vi "Make Deployable VI Path.vi"(1 "instance path":path) -> (0 "deployable path":path)   [LabVIEW 2020, in "NI_TargetHelper.lvlib"]
uses:
  <vilib>/TargetSupport/NI_TargetHelper/NI_TargetHelper.lvlib
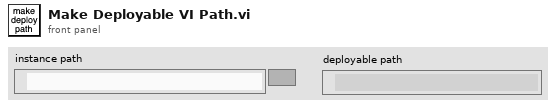
[diagram p1: front panel]
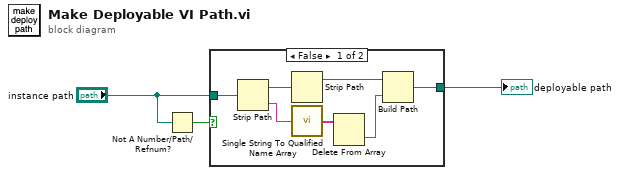
[diagram p0: block diagram]
diagram:
  n1 = Not A Number/Path/Refnum?(number/path/refnum="instance path") -> (NaN/Path/Refnum?=w2:bool)
  n2 = case shown="False" w2 {
    tunnel: "instance path" -> [w5 w11]
    tunnel: [w4 w11] -> w3
    frame False {
      n3 = Strip Path(path=w5) -> (stripped path=w7:path, name=w8:string)
      n4 = Strip Path(path=w7) -> (stripped path=w6:path)  [unwired: 1 out]
      n5 = call <vilib>:"Single String To Qualified Name Array.vi"("Fully Qualified String"=w8) -> ("Fully Qualified Array"=w10:string[])
      n6 = Delete From Array(array=w10) -> (deleted portion=w9:string)  [unwired: 2 in, 1 out]
      n7 = Build Path(base path=w6, name or relative path=w9) -> (appended path=w4:path)
    }
    frame True {
    }
  }
  "deployable path" <- w3
